vi "timestampInRange.vi"(10 "Time Stamp":timestamp, 11 "Start and end times":T1) -> (2 "timeState":T2(ring))   [LabVIEW 2017]
doc: "Check if given time stamp is before start, between start and end, or after end time."
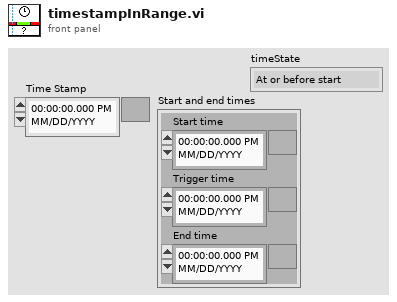
[diagram p1: front panel]
types:
  T1 = cluster{"Start time":timestamp, "Trigger time":timestamp, "End time":timestamp}
  T2 = enum16{"At or before start", "In range", "At or after end"}
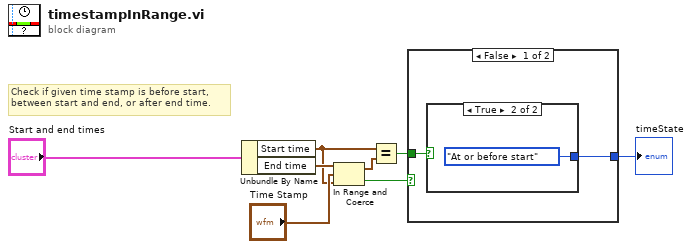
[diagram p0: block diagram]
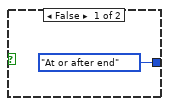
[diagram p2: hidden frame]
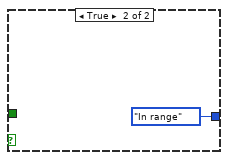
[diagram p3: hidden frame]
diagram:
  # "Check if given time stamp is before start, \nbetween start and end, or after end time."
  n1 = Unbundle By Name("Start and end times") -> ("Start time"=w6:timestamp, "End time"=w7:timestamp)
  n2 = In Range and Coerce(upper limit=w7, x="Time Stamp", lower limit=w6) -> (coerced(x)=w5:timestamp, In Range?=w4:bool)
  n3 = Equal?(x=w6, y=w5) -> (x = y?=w3:bool)
  n4 = case shown="False" w4 {
    tunnel: w3 -> [w10 _]
    tunnel: [w9 T2."In range"] -> w2
    frame False {
      n5 = case shown="True" w10 {
        tunnel: [T2."At or after end" T2."At or before start"] -> w9
        frame False {
        }
        frame True {
        }
      }
    }
    frame True {
    }
  }
  "timeState" <- w2
